vi "Configure Internal Trigger Rate [IT].vi"(8 "error in (no error)":errorcluster, 9 "trigger rate (0.0 trig/sec)":dbl[unit] format="%.3f", 11 "CS++Fgen in":refnum<class "CS++Fgen.lvclass">) -> (0 "error out":errorcluster, 3 "CS++Fgen out":refnum<class "CS++Fgen.lvclass">)   [LabVIEW 2013, in "CS++Fgen.lvlib" / "CS++Fgen.lvclass"]
doc: "This VI configures the rate at which the function generator's internal trigger source generates trigger signals.\n\nNotes:\n\n(1) This VI is part of the IviFgenInternalTrigger [IT] extension group."
uses:
  CS++Fgen.lvclass
  CSPP_Core/Classes/CS++ProcessVariables/ProcessVariable/PV.lvclass
  PV-Enum.ctl
  CSPP_Core/Classes/CS++ProcessVariables/ProcessVariable/PV.lvclass/PV.ctl
  CS++Fgen.lvclass/CS++Fgen.ctl
  CSPP_Core/Classes/CS++ProcessVariables/PVConnection/PVConnection.lvclass
  CSPP_Core/Classes/CS++ProcessVariables/ProcessVariable/Write Data.vi
  CSPP_Core/Classes/CS++ProcessVariables/ProcessVariable/Write Timestamp.vi
  CSPP_Core/Classes/CS++ProcessVariables/ProcessVariable/Write Quality.vi
  CSPP_Core/Classes/CS++ProcessVariables/ProcessVariable/Write status.vi
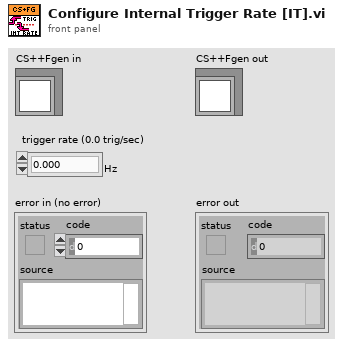
[diagram p1: front panel]
types:
  T1 = typedef "CS++Fgen.lvlib/CS++Fgen.lvclass/PV-Enum.ctl" = enum16{"AM-ModulationDepth", "AM-ModulationFrequency", "FM-ModulationFrequency", "FP-PeakDeviation", "SampleRate", "TriggerRate", "AM-ModulationWaveform", "FM-ModulationWaveform", "OutputMode", "ReferenceClockSource", "SampleClockSource", "SampleClockOutputEnabled"}
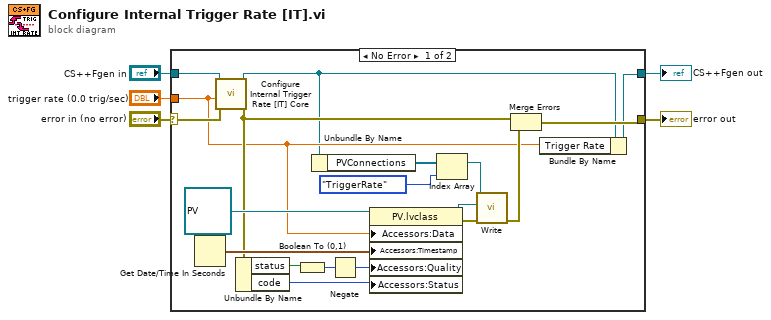
[diagram p0: block diagram]
diagram:
  n1 = case shown="No Error" "error in (no error)" {
    selector: "error in (no error)" -> [w23 w26]
    tunnel: [w11 w26] -> w4
    tunnel: [w9 w25] -> w2
    tunnel: "CS++Fgen in" -> [w24 w25]
    tunnel: "trigger rate (0.0 trig/sec)" -> [w12 _]
    frame No Error {
      n2 = Get Date/Time In Seconds() -> (seconds since 1Jan1904=w22:timestamp)
      n3 = call-dynamic "Configure Internal Trigger Rate [IT] Core.vi"("error in (no error)"=w23, "trigger rate (0.0 trig/sec)"=w12, "CS++Fgen in"=w24) -> ("error out"=w13:errorcluster, "CS++Fgen out"=w10:refnum<class "CS++Fgen.lvclass">)  [unwired: 7 in]
      n4 = Unbundle By Name(w13) -> ("status"=w17:bool, "code"=w15:i32)
      n5 = Boolean To (0,1)(Boolean=w17) -> (0, 1=w16:i16)
      n6 = Unbundle By Name(w10) -> ("PVConnections"=w8:refnum<class "PVConnection.lvclass">[])
      n7 = Negate(x=w16) -> (-x=w14:i16)
      n8 = property class="PV.lvclass"(reference=refnum<class "PV.lvclass"> refnum ("PV"), "Accessors:Data"=w12, "Accessors:Timestamp"=w22, "Accessors:Quality"=w14, "Accessors:Status"=w15) -> (reference out=w19:refnum<class "PV.lvclass">, error out=w20:errorcluster)  [unwired: 1 in]
      n9 = Index Array(array=w8, index=PV-Enum."TriggerRate" ("PV-Enum")) -> (element=w7:refnum<class "PVConnection.lvclass">)
      n10 = call-dynamic "Write.vi"("error in (no error)"=w20, "PV"=w19, "PVConnection in"=w7) -> ("error out"=w18:errorcluster)  [unwired: 7 in, 1 out]
      n11 = Merge Errors(w13, w18) -> (w11:errorcluster)
      n12 = Bundle By Name(cluster=w10, "Trigger Rate"=w12) -> (w9:refnum<class "CS++Fgen.lvclass">)
    }
    frame Error {
    }
  }
  "error out" <- w4
  "CS++Fgen out" <- w2
